vi "Wait for Child Safety.vi"(0 "GEA2 Reference In":refnum<k24>, 11 "Error In":errorcluster) -> (4 "GEA2 Reference Out":refnum<k24>, 6 "Pass/Fail?":bool, 8 "Report Text":string, 10 "Child Safety Duration (s)":dbl, 15 "Error Out":errorcluster)   [LabVIEW 2016, in "TL27.lvlib"]
doc: "Use this VI to wait for child safety complete."
uses:
  Projects/TL27.lvlib
  C:/Automation/DLLs/PC Dot Net/GeaCommunication.dll
  Common/LabVIEW GEA2 Toolkit/LabVIEW_GEA2_Toolkit.lvlibp/type defs/Source_Destination.ctl
  Common/LabVIEW GEA2 Toolkit/LabVIEW_GEA2_Toolkit.lvlibp/type defs/ERD Read Data In.ctl
  Common/LabVIEW GEA2 Toolkit/LabVIEW_GEA2_Toolkit.lvlibp/type defs/Data Type.ctl
  Common/LabVIEW GEA2 Toolkit/LabVIEW_GEA2_Toolkit.lvlibp
panel:
  in  "Standalone?":bool
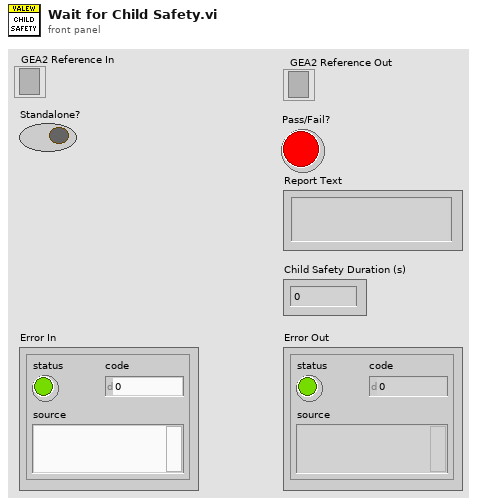
[diagram p1: front panel]
types:
  T1 = typedef "LabVIEW_GEA2_Toolkit.lvlibp/ERD Read Data In.ctl" = cluster{"ERD Number":u16, "Data Type":T2}
  T2 = typedef "LabVIEW_GEA2_Toolkit.lvlibp/Data Type.ctl" = enum16{"string", "boolean", "uint8_t", "uint16_t", "uint32_t", "uint64_t", "int8_t", "int16_t", "int32_t", "int64_t"}
  T3 = enum16{"EQ (==)", "NE (!=)", "GT (>)", "LT (<)", "GE (>=)", "LE (<=)", "GTLT(> <)", "GELE (>= <=)", "GELT (>= <)", "GTLE (> <=)", "LTGT (< >)", "LEGE (<= >=)", "LEGT (<= >)", "LTGE (< >=)", "No Comparison"}
  T4 = typedef "LabVIEW_GEA2_Toolkit.lvlibp/Source_Destination.ctl" = cluster{"Source":u8, "Destination":u8}
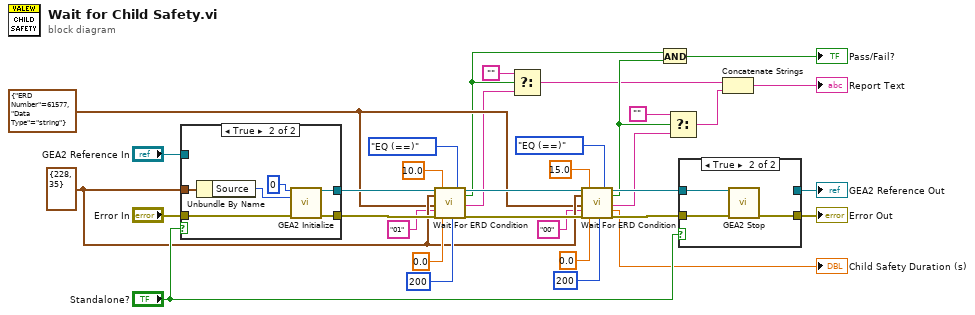
[diagram p0: block diagram]
diagram:
  w12 = T1 {"ERD Number"=61577, "Data Type"=enum."string"} ("ERD Read Data In")
  w13 = T4 {"Source"=228, "Destination"=35} ("GEA Inputs")
  n1 = case shown="True" "Standalone?" {
    tunnel: "Error In" -> [w35 w42]
    tunnel: [w35 w41] -> w14
    tunnel: "GEA2 Reference In" -> [w36 _]
    tunnel: [w36 w40] -> w15
    tunnel: w13 -> [_ w38]
    frame False {
    }
    frame True {
      n2 = Unbundle By Name(w38) -> ("Source"=w39:u8)
      n3 = call "GEA2 Initialize.vi"("Board Index"=0, "Source Address"=w39, "error in"=w42) -> ("GEA2 Reference Out"=w40:refnum<k24>, "error out"=w41:errorcluster)  [unwired: 10 in, 1 out]
    }
  }
  n4 = call "Wait For ERD Condition.vi"("GEA2 Reference In"=w15, "GEA Inputs"=w13, "ERD Read Data"=w12, "Expected Low"="01", "Error In"=w14, "Timeout (s)"=10.0, "Min Exec Time (s)"=0.0, "Loop Rate (ms)"=u32 200, "Comparison"=T3."EQ (==)") -> ("GEA2 Reference Out"=w17:refnum<k24>, "Pass/Fail?"=w8:bool, "Report Text"=w6:string, "Error Out"=w16:errorcluster)  [unwired: 6 in, 1 out]
  n5 = Select(t="", s=w8, f=w6) -> (s? t:f=w4:string)
  n6 = call "Wait For ERD Condition.vi"("GEA2 Reference In"=w17, "GEA Inputs"=w13, "ERD Read Data"=w12, "Expected Low"="00", "Error In"=w16, "Timeout (s)"=15.0, "Min Exec Time (s)"=0.0, "Loop Rate (ms)"=u32 200, "Comparison"=T3."EQ (==)") -> ("GEA2 Reference Out"=w29:refnum<k24>, "Pass/Fail?"=w5:bool, "Report Text"=w26:string, "Execution Time"=→"Child Safety Duration (s)":dbl, "Error Out"=w28:errorcluster)  [unwired: 6 in]
  n7 = And(x=w8, y=w5) -> (x .and. y?=→"Pass/Fail?":bool)
  n8 = Select(t="", s=w5, f=w26) -> (s? t:f=w3:string)
  n9 = case shown="True" "Standalone?" {
    tunnel: w28 -> [w44 w47]
    tunnel: [w44 w46] -> w34
    tunnel: [w43 _] -> w33
    tunnel: w29 -> [w43 w45]
    frame False {
    }
    frame True {
      n10 = call "GEA2 Stop.vi"("GEA2 Reference In"=w45, "Error In"=w47) -> ("Error Out"=w46:errorcluster)  [unwired: 13 in]
    }
  }
  "Error Out" <- w34
  "GEA2 Reference Out" <- w33
  n11 = Concatenate Strings(w4, w3) -> (→"Report Text":string)
